vi "KVMap-From String.vi"(7 "delimiter (Tab)":string=":", 11 "value":string) -> (3 "Cluster":cluster{string[], string[]})   [LabVIEW 2017]
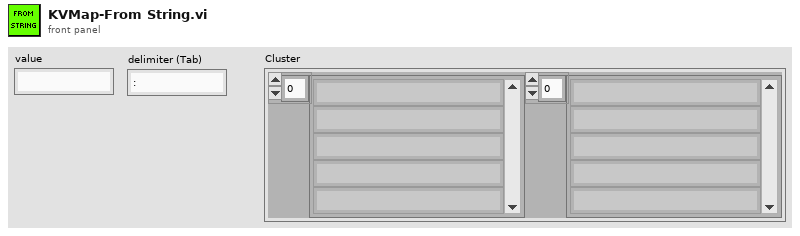
[diagram p1: front panel]
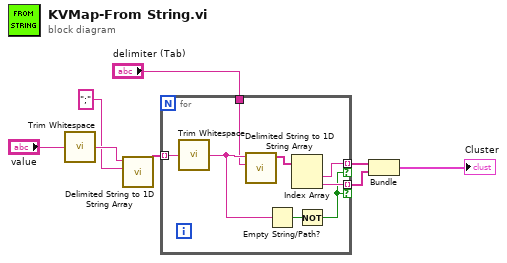
[diagram p0: block diagram]
diagram:
  n1 = call-poly <vilib>:"Trim Whitespace.vi"("string"="value") -> ("trimmed string"=w2:string)  [unwired: 1 in]
  n2 = call "Delimited String to 1D String Array.vi"("delimiter"=";" ("delimiter (Tab)"), "delimited string"=w2) -> ("string array"=w5:string[])  [unwired: 9 in]
  n3 = for {
    tunnel: w5 -> [w13] mode=indexing
    tunnel: [w15] -> w6 mode=indexing if=w11
    tunnel: [w14] -> w7 mode=indexing if=w11
    tunnel: "delimiter (Tab)" -> [w9]
    n4 = call-poly <vilib>:"Trim Whitespace.vi"("string"=w13) -> ("trimmed string"=w10:string)  [unwired: 1 in]
    n5 = call "Delimited String to 1D String Array.vi"("delimiter"=w9, "delimited string"=w10) -> ("string array"=w16:string[])  [unwired: 9 in]
    n6 = Empty String/Path?(string/path=w10) -> (empty?=w12:bool)
    n7 = Index Array(array=w16) -> (element #1=w15:string, element #2=w14:string)  [unwired: 2 in]
    n8 = Not(x=w12) -> (.not. x?=w11:bool)
  }
  n9 = Bundle(w6, w7) -> (→"Cluster":cluster{string[], string[]})  [unwired: 1 in]
